vi "photocell.vi"() -> ()   [LabVIEW 2013]
uses:
  <vilib>/LabVIEW Interface for Arduino/Type Defs/Pin Mode.ctl
  <vilib>/LabVIEW Interface for Arduino/LabVIEW Interface for Arduino.lvlib
panel:
  out "0, 1":i16
  out "Waveform Chart":dbl(graph)
  in  "Digital I/O Pin (0)":u8
  in  "millisecond multiple":u32=300
  in  "Analog Input Pin (0)":u8
  in  "stop":bool
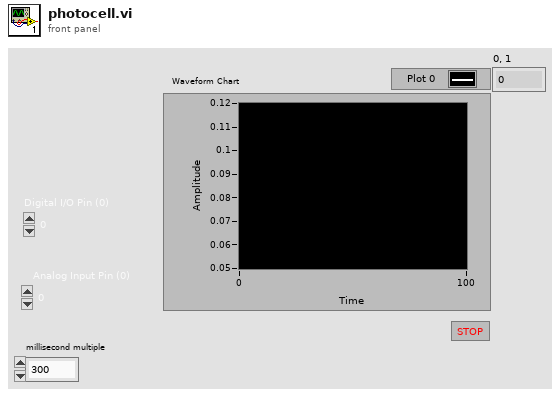
[diagram p1: front panel]
types:
  T1 = typedef "LabVIEW Interface for Arduino.lvlib/Pin Mode.ctl" = enum8{"Input", "Output"}
  T2 = typedef "LabVIEW Interface for Arduino.lvlib/Arduino Resource.ctl" = cluster{"VISA resource":refnum<visa-resource-name>, "Board Type":T3, "Connection Type":enum8{"USB / Serial"}, "Bytes Per Packet (15)":u8}
  T3 = typedef "LabVIEW Interface for Arduino.lvlib/Board Type.ctl" = enum16{"Uno", "Dimuelanove w/Atmega 328", "Mega 2560"}
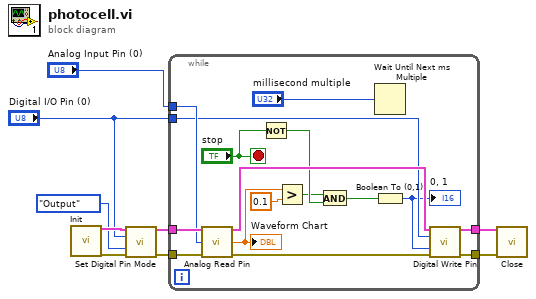
[diagram p0: block diagram]
diagram:
  n1 = call <vilib>:"Init.vi"() -> ("Arduino Resource"=w4:T2, "error out"=w6:errorcluster)  [unwired: 18 in]
  n2 = call <vilib>:"Set Digital Pin Mode.vi"("Arduino Resource"=w4, "Digital I/O Pin"="Digital I/O Pin (0)", "Pin Mode (Input)"=Pin_Mode."Output", "error in"=w6) -> ("Arduino Resource"=w3:T2, "error out"=w5:errorcluster)  [unwired: 10 in]
  n3 = while {
    tunnel: "Analog Input Pin (0)" -> [w18]
    tunnel: [w24] -> w8
    tunnel: [w23] -> w7
    tunnel: w5 -> [w22]
    tunnel: w3 -> [w20]
    tunnel: "Digital I/O Pin (0)" -> [w17]
    stop <- "stop" stop-if-true
    n4 = call <vilib>:"Analog Read Pin.vi"("Arduino Resource"=w20, "Analog Input Pin (0)"=w18, "error in"=w22) -> ("Arduino Resource"=w19:T2, "Voltage"=w14:dbl, "error out"=w21:errorcluster)  [unwired: 10 in]
    "Waveform Chart" <- w14
    n5 = Not(x="stop") -> (.not. x?=w12:bool)
    n6 = Greater?(x=w14, y=0.1) -> (0:w11:bool)
    n7 = And(x=w11, y=w12) -> (x .and. y?=w10:bool)
    n8 = Wait Until Next ms Multiple(millisecond multiple="millisecond multiple") -> ()  [unwired: 1 out]
    n9 = Boolean To (0,1)(Boolean=w10) -> (0, 1=w15:i16)
    "0, 1" <- w15
    n10 = call <vilib>:"Digital Write Pin.vi"("Arduino Resource"=w19, "Digital I/O Pin (0)"=w17, "Value (0)"=w15, "error in"=w21) -> ("Arduino Resource"=w23:T2, "error out"=w24:errorcluster)  [unwired: 10 in]
  }
  n11 = call <vilib>:"Close.vi"("Arduino Resource"=w7, "error in"=w8) -> ()  [unwired: 13 in, 1 out]
